vi "Read action name.vi"(8 "error in (no error)":errorcluster, 11 "RenameVIsandClasses in":refnum<class "SequencerActionScript.lvclass">) -> (0 "error out":errorcluster, 2 "action name":string, 3 "RenameVIsandClasses out":refnum<class "SequencerActionScript.lvclass">)   [LabVIEW 2014, in "SequencerActionScript.lvclass"]
uses:
  SequencerActionScript.lvclass
  SequencerActionScript.lvclass/SequencerActionScript.ctl
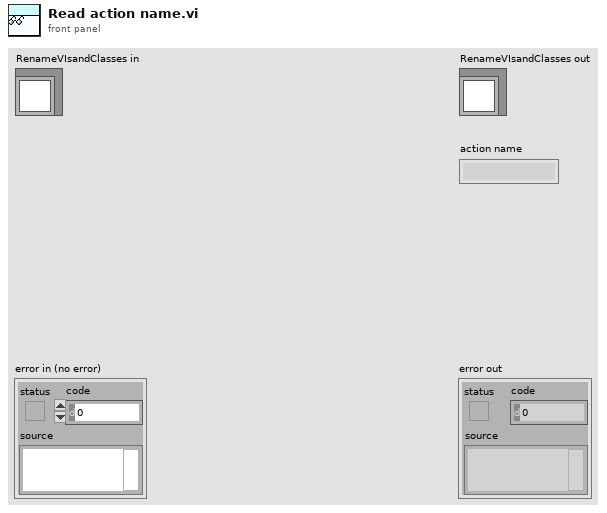
[diagram p1: front panel]
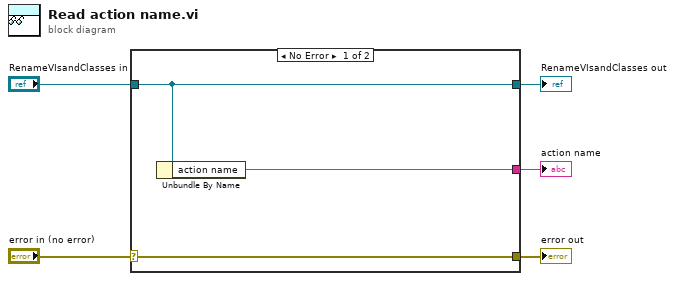
[diagram p0: block diagram]
diagram:
  n1 = case shown="No Error" "error in (no error)" {
    selector: "error in (no error)" -> [w8 w9]
    tunnel: [w8 w9] -> w4
    tunnel: [w7 w10] -> w2
    tunnel: "RenameVIsandClasses in" -> [w7 w10]
    tunnel: [w6 _] -> w1
    frame No Error {
      n2 = Unbundle By Name(w7) -> ("action name"=w6:string)
    }
    frame Error {
    }
  }
  "error out" <- w4
  "RenameVIsandClasses out" <- w2
  "action name" <- w1
